vi "SMUSineWithReferenceTrigger.vi"() -> ()   [LabVIEW 2024]
uses:
  <instrlib>/niScope/Controls/niScope vertical coupling.ctl
  <instrlib>/niDCPower/nidcpower.llb/niDCPower Output Function.ctl
  <instrlib>/niDCPower/nidcpower.llb/niDCPower Source Mode.ctl
  <instrlib>/niDCPower/nidcpower.llb/niDCPower Export Signal - Signal.ctl
  <instrlib>/niScope/Controls/niScope trigger source digital.ctl
  <instrlib>/niScope/Controls/niScope trigger slope.ctl
  <instrlib>/niScope/Configure/Trigger/niScope Configure Trigger Digital.vi
  <instrlib>/niScope/Measurements/niScope Fetch Array Measurement Cluster.vi
panel:
  out "SMU Current":cluster{dbl, dbl}[](graph)
  out "Scope Waveform":T1(graph)
  in  "Configure":enum32{"SMU", "Scope"}(tab)
  in  "SMUname":refnum<k15> caption="resource name"
  in  "?":enum32{"Standard Transients", "Custom"}(tab)
  in  "Source:Transient Response":i32(ring)=1039 items=["Slow"=1041, "Normal"=1038, "Fast"=1039, "Custom"=1042]
  in  "Gain Bandwidth":dbl=5000.0
  in  "Pole-Zero Ratio":dbl=0.16
  in  "Compensation Frequency":dbl=50000.0
  in  "Stimulus Type":enum32{"Sine", "Square"}(tab)
  in  "Amplitude":dbl=2.0
  in  "Frequency":dbl=1000.0 format="%#_6p"
  in  "Samples per Sine":u16=20
  in  "DC offset":dbl=1.0
  in  "LowLevel":dbl=1.0
  in  "HighLevel":dbl=2.0
  in  "OnTime":dbl=5e-06 format="%#_6p"
  in  "Signal Duration":u32=2
  in  "Fixed Source Delay":dbl=2e-06 format="%#_6p"
  out "Apperature Time":dbl format="%#_6p"
  in  "SMU Function":T2=1007 items=["DC Voltage"=1006, "DC Current"=1007, "Pulse Voltage"=1049, "Pulse Current"=1050]
  in  "DC Source Limit":dbl=20.0
  in  "resource name":refnum<k15> caption="Scope Name"
  in  "vertical coupling":T3=1 items=["AC", "DC", "Ground"]
  in  "channels":string="0"
  out "Stimulus In":cluster{dbl, dbl}[](graph)
  out "SMU Voltage":cluster{dbl, dbl}[](graph)
  out "error out":errorcluster
  # "Only DC Current or Voltage"
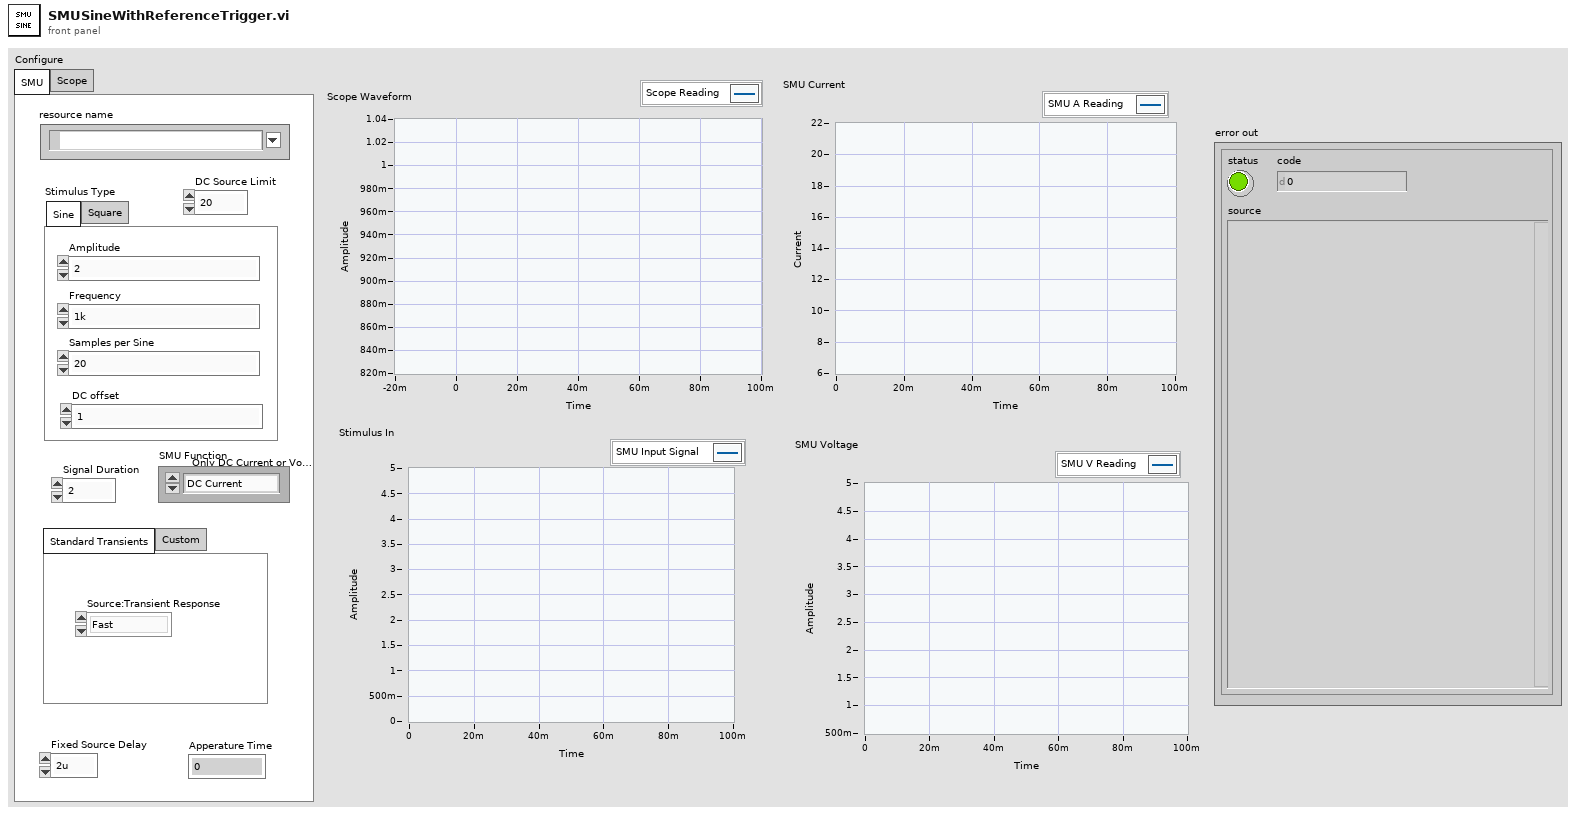
[diagram p1: front panel]
types:
  T1 = cluster{"relativeInitialX":dbl, "xIncrement":dbl, "measWfm":dbl[]}
  T2 = typedef "niDCPower Output Function.ctl" = i32
  T3 = typedef "niScope vertical coupling.ctl" = i32
  T4 = typedef "niDCPower Export Signal - Signal.ctl" = i32
  T5 = typedef "niDCPower Source Mode.ctl" = i32
  T6 = typedef "niScope trigger source digital.ctl" = string
  T7 = typedef "niScope trigger slope.ctl" = i32
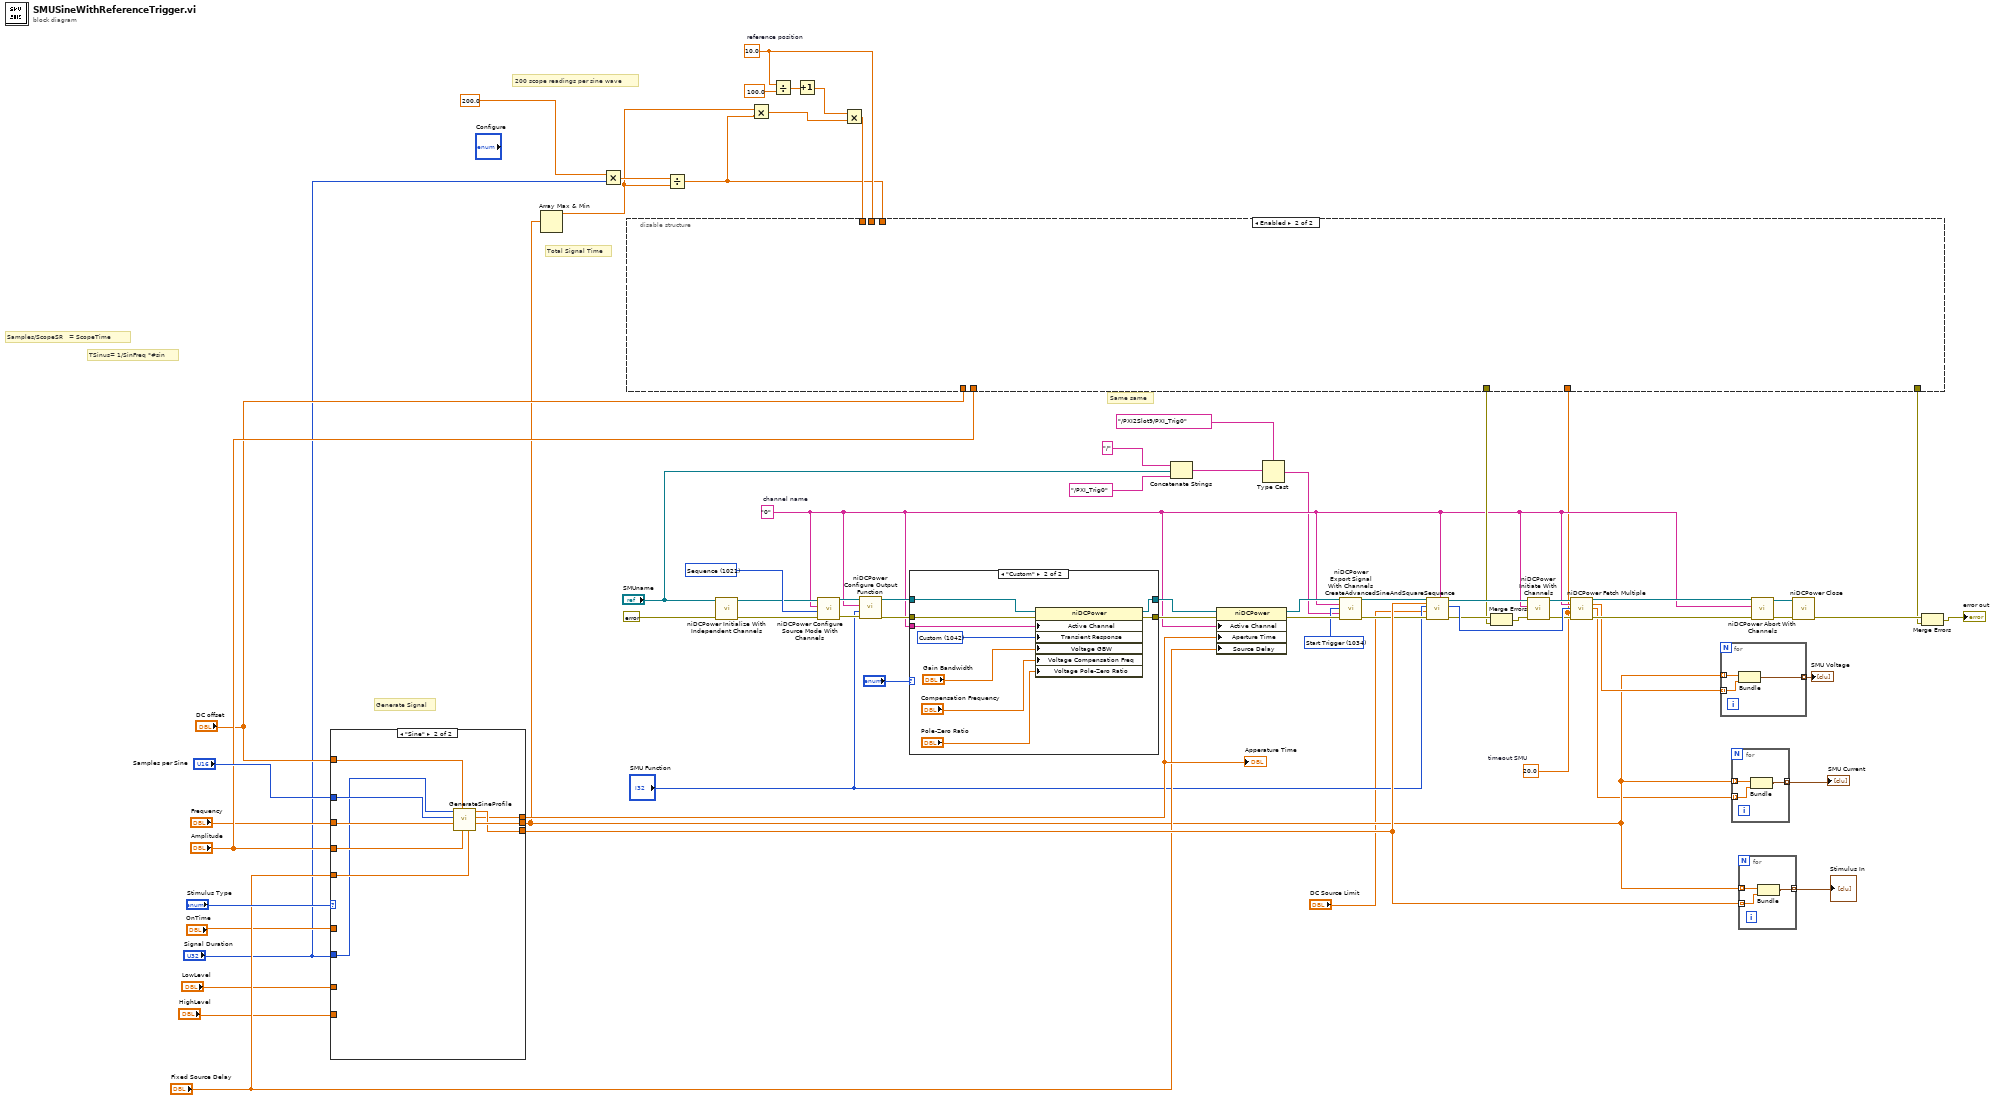
[diagram p0: block diagram]
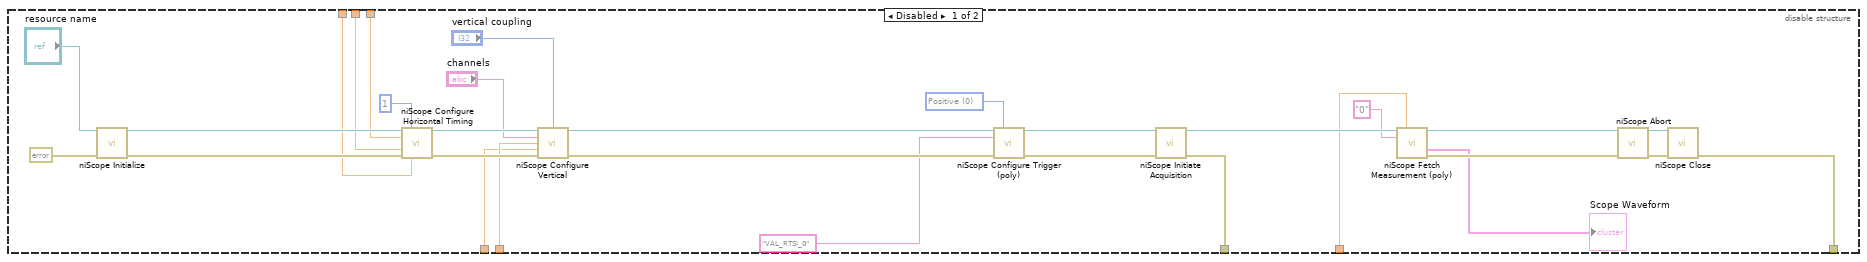
[diagram p2: hidden frame]
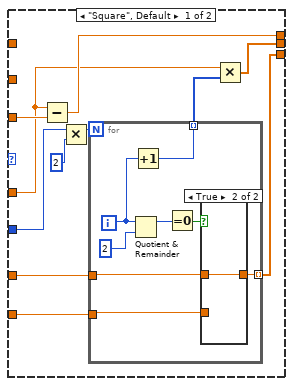
[diagram p3: hidden frame]
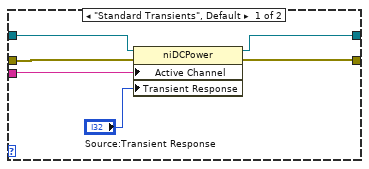
[diagram p5: hidden frame]
diagram:
  w30 = T4 1034 items=["Source Complete Event"=1030, "Measure Complete Event"=1031, "Sequence Iteration Complete Event"=1032, "Sequence Engine Done Event"=1033, "Pulse Complete Event"=1051, "Ready For Pulse Trigger Event"=1052, "Start Trigger"=1034, "Source Trigger"=1035, "Measure Trigger"=1036, "Sequence Advance Trigger"=1037, "Pulse Trigger"=1053] ("signal")
  w22 = 10.0  # reference position
  w29 = 20.0  # timeout SMU
  w61 = T5 1021 items=["Single Point"=1020, "Sequence"=1021] ("source mode")
  w31 = "0"  # channel name
  # "Generate Signal"
  # "Total Signal Time"
  # "200 scope readings per sine wave"
  # "Samples/ScopeSR   = ScopeTime"
  # "TSinus= 1/SinFreq *#sin"
  # "Same same"
  n1 = case shown="\"Sine\"" "Stimulus Type" {
    tunnel: "Samples per Sine" -> [_ w98]
    tunnel: [w69 w97] -> w4
    tunnel: [w72 w96] -> w49
    tunnel: [w78 w95] -> w46
    tunnel: "Fixed Source Delay" -> [w79 w94]
    tunnel: "Amplitude" -> [_ w93]
    tunnel: "DC offset" -> [_ w92]
    tunnel: "Frequency" -> [_ w91]
    tunnel: "OnTime" -> [w70 _]
    tunnel: "Signal Duration" -> [w75 w90]
    tunnel: "LowLevel" -> [w77 _]
    tunnel: "HighLevel" -> [w76 _]
    frame "Square", Default {
      n2 = Subtract(x=w70, y=w79) -> (x-y=w78:dbl)
      n3 = Multiply(x=w75, y=u32 2) -> (x*y=w74:u32)
      n4 = for {
        N: w74 -> [_]
        tunnel: w77 -> [w83]
        tunnel: w76 -> [w82]
        tunnel: [w84] -> w72 mode=indexing
        tunnel: [w80] -> w71 mode=indexing
        i -> [w81]
        n5 = Quotient & Remainder(x=w81, y=2) -> (x-y*floor(x/y)=w86:i32)  [unwired: 1 out]
        n6 = Increment(x=w81) -> (x+1=w80:i32)
        n7 = Equal To 0?(x=w86) -> (x = 0?=w85:bool)
        n8 = case shown="True" w85 {
          tunnel: [w88 w89] -> w84
          tunnel: w83 -> [_ w89]
          tunnel: w82 -> [w88 _]
          frame False {
          }
          frame True {
          }
        }
      }
      n9 = Multiply(x=w70, y=w71) -> (x*y=w69:dbl[])
    }
    frame "Sine" {
      n10 = call "GenerateSineProfile.vi"("Fixed Source Delay of"=w94, "Amplitude"=w93, "DC offset"=w92, "Frequency"=w91, "Samples per Sine"=w98, "Amount of Itterations"=w90) -> ("Time to Plot"=w97:dbl[], "Apperature Time"=w95:dbl, "Voltage"=w96:dbl[])  [unwired: 3 in]
    }
  }
  "Apperature Time" <- w46
  n11 = Array Max & Min(array=w4) -> (max value=w6:dbl)  [unwired: 3 out]
  n12 = Multiply(x=200.0 ("y"), y="Signal Duration") -> (x*y=w8:dbl)
  n13 = Divide(x=w8, y=w6) -> (x/y=w7:dbl)
  n14 = call <instrlib>:"niDCPower Initialize With Independent Channels.vi"("error in (no error)"=errorcluster {"status"=FALSE, "code"=0, "source"=""}, "resource name"="SMUname") -> ("error out"=w59:errorcluster, "instrument handle out"=w60:refnum<k15>)  [unwired: 8 in]
  n15 = Multiply(x=w6, y=w7) -> (x*y=w16:dbl)
  n16 = Divide(x=w22, y=100.0) -> (x/y=w20:dbl)
  n17 = Increment(x=w20) -> (x+1=w19:dbl)
  n18 = call <instrlib>:"niDCPower Configure Source Mode With Channels.vi"("error in (no error)"=w59, "source mode"=w61, "channel name"=w31, "instrument handle"=w60) -> ("error out"=w57:errorcluster, "instrument handle out"=w58:refnum<k15>)  [unwired: 6 in]
  n19 = Multiply(x=w19, y=w16) -> (x*y=w18:dbl)
  n20 = disable-structure shown="Enabled" {
    disable-tunnel: [w116 _] -> w42
    disable-tunnel: [w114 _] -> w39
    disable-tunnel: "Amplitude" -> [w110 _]
    disable-tunnel: "DC offset" -> [w109 _]
    disable-tunnel: w29 -> [w105 _]
    disable-tunnel: w22 -> [w102 _]
    disable-tunnel: w18 -> [w101 _]
    disable-tunnel: w7 -> [w99 _]
    frame Disabled {
      w106 = T7 0 items=["Positive", "Negative"] ("trigger slope")
      n21 = call <instrlib>:"niScope Initialize.vi"("resource name"="resource name", "error in"=errorcluster {"status"=FALSE, "code"=0, "source"=""}) -> ("instrument handle"=w129:refnum<k15>, "error out"=w128:errorcluster)  [unwired: 12 in]
      n22 = call <instrlib>:"niScope Configure Horizontal Timing.vi"("instrument handle"=w129, "number of records"=1, "min sample rate"=w99, "reference position"=w102, "error in"=w128, "min record length"=w101) -> ("instrument handle out"=w127:refnum<k15>, "error out"=w126:errorcluster)  [unwired: 8 in]
      n23 = call <instrlib>:"niScope Configure Vertical.vi"("instrument handle"=w127, "vertical coupling"="vertical coupling", "channels"="channels", "vertical range"=w110, "vertical offset"=w109, "error in"=w126) -> ("instrument handle out"=w125:refnum<k15>, "error out"=w124:errorcluster)  [unwired: 8 in]
      n24 = call-poly <instrlib>:"niScope Configure Trigger (poly).vi"("instrument handle"=w125, "trigger slope"=w106, "trigger source"=T6 "VAL_RTSI_0", "error in"=w124) -> ("instrument handle out"=w123:refnum<k15>, "error out"=w122:errorcluster)  [unwired: 10 in]
      n25 = call <instrlib>:"niScope Initiate Acquisition.vi"("instrument handle"=w123, "error in"=w122) -> ("instrument handle out"=w121:refnum<k15>, "error out"=w116:errorcluster)  [unwired: 12 in]
      n26 = call-poly <instrlib>:"niScope Fetch Measurement (poly).vi"("instrument handle"=w121, "timeout"=w105, "channels"="0") -> ("instrument handle out"=w120:refnum<k15>, "meas waveform"=→"Scope Waveform":T1, "error in"=w115:errorcluster, "error out"=w119:errorcluster)  [unwired: 8 in, 1 out]
      n27 = call <instrlib>:"niScope Abort.vi"("instrument handle"=w120, "error in"=w119) -> ("instrument handle out"=w118:refnum<k15>, "error out"=w117:errorcluster)  [unwired: 12 in]
      n28 = call <instrlib>:"niScope Close.vi"("instrument handle"=w118, "error in"=w117) -> ("error out"=w114:errorcluster)  [unwired: 13 in]
    }
    frame Enabled {
    }
  }
  n29 = call <instrlib>:"niDCPower Configure Output Function.vi"("error in (no error)"=w57, "output function"="SMU Function", "channel name"=w31, "instrument handle"=w58) -> ("error out"=w55:errorcluster, "instrument handle out"=w54:refnum<k15>)  [unwired: 6 in]
  n30 = case shown="\"Custom\"" "?" {
    tunnel: [w135 w144] -> w47
    tunnel: w55 -> [w132 w143]
    tunnel: w54 -> [w133 w142]
    tunnel: w31 -> [w131 w141]
    tunnel: [w134 w140] -> w48
    frame "Standard Transients", Default {
      n31 = property class="niDCPower"(reference=w133, error in=w132, "Active Channel"=w131, "Transient Response"="Source:Transient Response") -> (reference out=w134:refnum<k15>, error out=w135:errorcluster)
    }
    frame "Custom" {
      w139 = 1042 items=["Slow"=1041, "Normal"=1038, "Fast"=1039, "Custom"=1042] ("Source:Transient Response")
      n32 = property class="niDCPower"(reference=w142, error in=w143, "Active Channel"=w141, "Transient Response"=w139, "Voltage GBW"="Gain Bandwidth", "Voltage Compensation Freq"="Compensation Frequency", "Voltage Pole-Zero Ratio"="Pole-Zero Ratio") -> (reference out=w140:refnum<k15>, error out=w144:errorcluster)
    }
  }
  n33 = Concatenate Strings("/" ("string"), "SMUname", "/PXI_Trig0" ("string")) -> (w24:string)
  n34 = property class="niDCPower"(reference=w48, error in=w47, "Active Channel"=w31, "Aperture Time"=w46, "Source Delay"="Fixed Source Delay") -> (reference out=w33:refnum<k15>, error out=w35:errorcluster)
  n35 = Type Cast(type=tag "/PXI2Slot9/PXI_Trig0" ("output terminal"), x=w24) -> (*(type *) &x=w28:tag)
  n36 = call <instrlib>:"niDCPower Export Signal With Channels.vi"("instrument handle"=w33, "channel name"=w31, "signal"=w30, "output terminal"=w28, "error in (no error)"=w35) -> ("instrument handle out"=w32:refnum<k15>, "error out"=w34:errorcluster)  [unwired: 9 in]
  n37 = call "CreateAdvancedSineAndSquareSequence.vi"("channel name"=w31, "Stimulus Profile"=w49, "error in (no error)"=w34, "DC Source Limit"="DC Source Limit", "Output Function"="SMU Function", "IVI Refnum in"=w32) -> ("error out"=w43:errorcluster, "Numbers of Samples to Read"=w56:i32, "IVI Refnum out"=w66:refnum<k15>)  [unwired: 3 in]
  n38 = Merge Errors(w43, w42) -> (w44:errorcluster)
  n39 = call <instrlib>:"niDCPower Initiate With Channels.vi"("error in (no error)"=w44, "channel name"=w31, "instrument handle"=w66) -> ("error out"=w41:errorcluster, "instrument handle out"=w65:refnum<k15>)  [unwired: 7 in]
  n40 = call <instrlib>:"niDCPower Fetch Multiple.vi"("instrument handle"=w65, "channel name"=w31, "count (1)"=w56, "timeout (1.0)"=w29, "error in (no error)"=w41) -> ("instrument handle out"=w68:refnum<k15>, "voltage measurements"=w52:dbl[], "current measurements"=w3:dbl[], "error out"=w67:errorcluster)  [unwired: 5 in, 2 out]
  n41 = for {
    tunnel: w4 -> [w147] mode=indexing
    tunnel: w52 -> [w146] mode=indexing
    tunnel: [w145] -> w51 mode=indexing
    n42 = Bundle(w147, w146) -> (w145:cluster{dbl, dbl})  [unwired: 1 in]
  }
  "SMU Voltage" <- w51
  n43 = for {
    tunnel: w4 -> [w150] mode=indexing
    tunnel: w3 -> [w149] mode=indexing
    tunnel: [w148] -> w2 mode=indexing
    n44 = Bundle(w150, w149) -> (w148:cluster{dbl, dbl})  [unwired: 1 in]
  }
  "SMU Current" <- w2
  n45 = for {
    tunnel: w4 -> [w153] mode=indexing
    tunnel: w49 -> [w152] mode=indexing
    tunnel: [w151] -> w50 mode=indexing
    n46 = Bundle(w153, "LowLevel"=w152) -> (w151:cluster{dbl, "LowLevel":dbl})  [unwired: 1 in]
  }
  "Stimulus In" <- w50
  n47 = call <instrlib>:"niDCPower Abort With Channels.vi"("error in (no error)"=w67, "channel name"=w31, "instrument handle"=w68) -> ("error out"=w63:errorcluster, "instrument handle out"=w64:refnum<k15>)  [unwired: 7 in]
  n48 = call <instrlib>:"niDCPower Close.vi"("error in (no error)"=w63, "instrument handle"=w64) -> ("error out"=w40:errorcluster)  [unwired: 9 in]
  n49 = Merge Errors(w40, w39) -> (→"error out":errorcluster)
